vi "Add content to Engine library.vi"(6 "Project Name":string, 8 "error in (no error)":errorcluster, 9 "Project Root":path, 10 "CD Wizard - Internal Data":T1, 11 "Inline-Async":refnum<class "NIVS_Inline HW Interface (Inline-Async).lvclass">) -> (0 "error out":errorcluster)   [LabVIEW 2015, in "NIVS_Inline HW Interface (Inline-Async).lvclass"]
doc: "Add all virtual folders and VIs to the Engine library."
uses:
  NIVS_Inline HW Interface (Inline-Async).lvclass
  NIVS_Consolidated_CDW_MetaDataObj/Internal data.ctl
  NIVS_Consolidated_CDW_MetaDataObj/CD Engine lvlib.ctl
  NIVS_Consolidated_CDW_MetaDataObj/Add Item - Type.ctl
  NIVS_Consolidated_CDW_MetaDataObj/CD Engine lvlib.vi
  NIVS_Consolidated_CDW_MetaDataObj/NIVS_Consolidated_CDW_MetaDataObj.lvclass
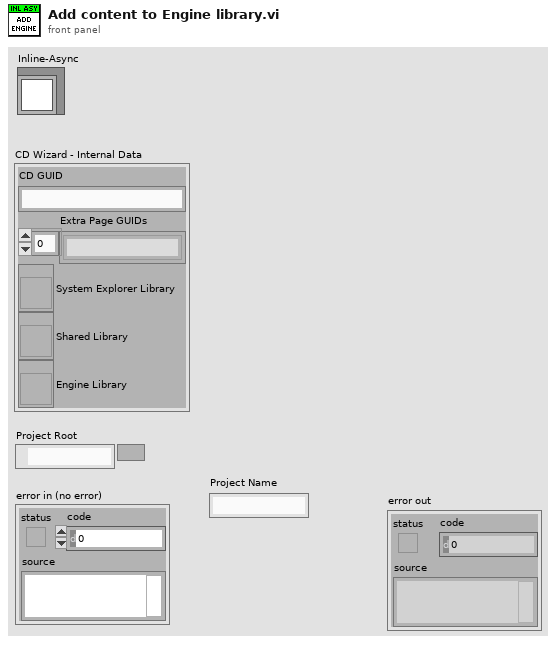
[diagram p1: front panel]
types:
  T1 = typedef "NIVS_Consolidated_CDW_MetaDataObj.lvclass/Internal data.ctl" = cluster{"CD GUID":string, "Extra Page GUIDs":string[], "System Explorer Library":refnum<vi>, "Shared Library":refnum<vi>, "Engine Library":refnum<vi>}
  T2 = typedef "NIVS_Consolidated_CDW_MetaDataObj.lvclass/CD Engine lvlib.ctl" = enum16{"LibraryFileName", "LibraryFolderName", "Engine.FolderName", "Engine.Init.FolderName", "Engine.Run.FolderName", "Engine.Shutdown.FolderName", "Types.FolderName", "Engine.RT Driver VI.TemplatePath", "Engine.RT Driver VI.FileName", "Engine.RTStateVariables.Name", "Engine.RTStateVariables.Name.NoExtension", "Engine.Async.NameExtension", "Engine.Async.TemplateName"}
  T3 = typedef "NIVS_Consolidated_CDW_MetaDataObj.lvclass/Add Item - Type.ctl" = string
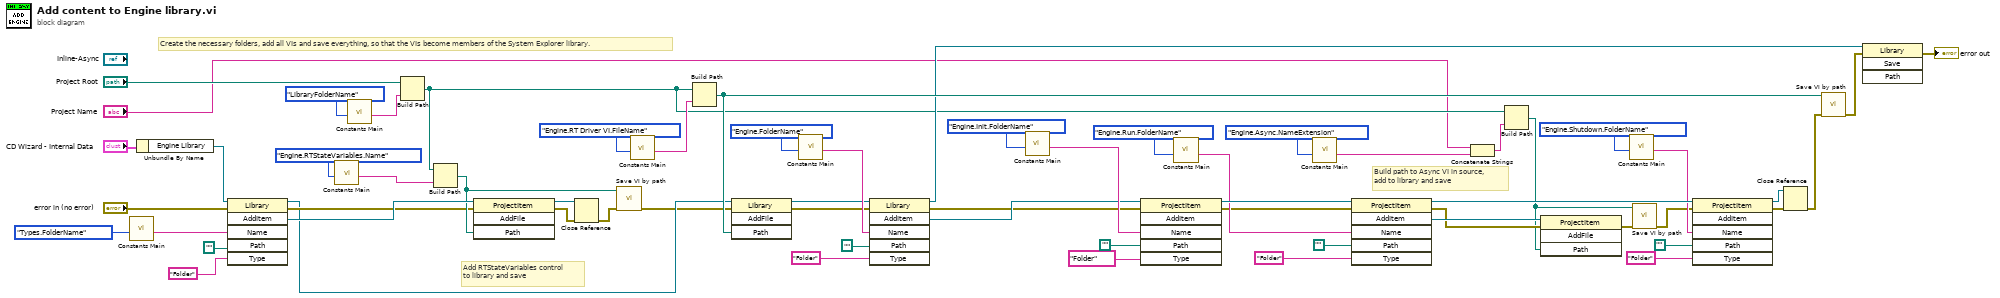
[diagram p0: block diagram]
diagram:
  # "Create the necessary folders, add all VIs and save everything, so that the VIs become members of the System Explorer library."
  # "Add RTStateVariables control\nto library and save"
  # "Build path to Async VI in source,\nadd to library and save"
  n1 = call-poly "Constants Main.vi"("Action"=CD_Engine_lvlib."Types.FolderName") -> ("Output"=w58:string)  [unwired: 10 in]
  n2 = Unbundle By Name("CD Wizard - Internal Data") -> ("Engine Library"=w48:refnum<vi>)
  n3 = invoke class="Library" method="AddItem"(reference=w48, error in="error in (no error)", "Name"=w58, "Path"=path "", "Type"=T3 "Folder" ("Add Item - Type")) -> (reference out=w9:refnum<vi>, error out=w10:errorcluster, "AddItem"=w25:refnum<vi>)  [unwired: 1 in, 3 out]
  n4 = call-poly "Constants Main.vi"("Action"=CD_Engine_lvlib."Engine.RTStateVariables.Name") -> ("Output"=w13:string)  [unwired: 10 in]
  n5 = call-poly "Constants Main.vi"("Action"=CD_Engine_lvlib."LibraryFolderName") -> ("Output"=w50:string)  [unwired: 10 in]
  n6 = Build Path(base path="Project Root", name or relative path=w50) -> (appended path=w20:path)
  n7 = Build Path(base path=w20, name or relative path=w13) -> (appended path=w23:path)
  n8 = invoke class="ProjectItem" method="AddFile"(reference=w25, error in=w10, "Path"=w23) -> (reference out=w5:refnum<vi>, error out=w24:errorcluster)  [unwired: 1 in, 2 out]
  n9 = Close Reference(reference=w5, error in (no error)=w24) -> (error out=w6:errorcluster)
  n10 = call "Save VI by path.vi"("error in (no error)"=w6, "VI path"=w23) -> ("error out"=w8:errorcluster)  [unwired: 9 in]
  n11 = call-poly "Constants Main.vi"("Action"=CD_Engine_lvlib."Engine.RT Driver VI.FileName") -> ("Output"=w52:string)  [unwired: 10 in]
  n12 = Build Path(base path=w20, name or relative path=w52) -> (appended path=w31:path)
  n13 = invoke class="Library" method="AddFile"(reference=w9, error in=w8, "Path"=w31) -> (reference out=w43:refnum<vi>, error out=w7:errorcluster)  [unwired: 1 in, 2 out]
  n14 = call-poly "Constants Main.vi"("Action"=CD_Engine_lvlib."Engine.FolderName") -> ("Output"=w45:string)  [unwired: 10 in]
  n15 = invoke class="Library" method="AddItem"(reference=w43, error in=w7, "Name"=w45, "Path"=path "", "Type"=T3 "Folder" ("Add Item - Type")) -> (reference out=w30:refnum<vi>, error out=w4:errorcluster, "AddItem"=w42:refnum<vi>)  [unwired: 1 in, 3 out]
  n16 = call-poly "Constants Main.vi"("Action"=CD_Engine_lvlib."Engine.Init.FolderName") -> ("Output"=w54:string)  [unwired: 10 in]
  n17 = invoke class="ProjectItem" method="AddItem"(reference=w42, error in=w4, "Name"=w54, "Path"=path "", "Type"=T3 "Folder" ("Add Item - Type")) -> (reference out=w40:refnum<vi>, error out=w3:errorcluster)  [unwired: 1 in, 4 out]
  n18 = call-poly "Constants Main.vi"("Action"=CD_Engine_lvlib."Engine.Run.FolderName") -> ("Output"=w38:string)  [unwired: 10 in]
  n19 = call-poly "Constants Main.vi"("Action"=CD_Engine_lvlib."Engine.Async.NameExtension") -> ("Output"=w15:string)  [unwired: 10 in]
  n20 = invoke class="ProjectItem" method="AddItem"(reference=w40, error in=w3, "Name"=w38, "Path"=path "", "Type"=T3 "Folder" ("Add Item - Type")) -> (reference out=w32:refnum<vi>, error out=w19:errorcluster, "AddItem"=w22:refnum<vi>)  [unwired: 1 in, 3 out]
  n21 = Concatenate Strings("Project Name", w15) -> (w21:string)
  n22 = Build Path(base path=w20, name or relative path=w21) -> (appended path=w17:path)
  n23 = invoke class="ProjectItem" method="AddFile"(reference=w22, error in=w19, "Path"=w17) -> (error out=w18:errorcluster)  [unwired: 1 in, 3 out]
  n24 = call-poly "Constants Main.vi"("Action"=CD_Engine_lvlib."Engine.Shutdown.FolderName") -> ("Output"=w29:string)  [unwired: 10 in]
  n25 = call "Save VI by path.vi"("error in (no error)"=w18, "VI path"=w17) -> ("error out"=w2:errorcluster)  [unwired: 9 in]
  n26 = invoke class="ProjectItem" method="AddItem"(reference=w32, error in=w2, "Name"=w29, "Path"=path "", "Type"=T3 "Folder" ("Add Item - Type")) -> (reference out=w26:refnum<vi>, error out=w28:errorcluster)  [unwired: 1 in, 4 out]
  n27 = Close Reference(reference=w26, error in (no error)=w28) -> (error out=w27:errorcluster)
  n28 = call "Save VI by path.vi"("error in (no error)"=w27, "VI path"=w31) -> ("error out"=w60:errorcluster)  [unwired: 9 in]
  n29 = invoke class="Library" method="Save"(reference=w30, error in=w60) -> (error out=→"error out":errorcluster)  [unwired: 2 in, 3 out]
